vi "Setup TS.vi"(8 "error in":errorcluster, 11 "Water Tunnel Test Stand in":refnum<class "Water Tunnel Test Stand.lvclass">) -> (0 "error out":errorcluster, 3 "Water Tunnel Test Stand out":refnum<class "Water Tunnel Test Stand.lvclass">)   [LabVIEW 2019, in "Test Stands.lvlib" / "Water Tunnel Test Stand.lvclass"]
uses:
  Water Tunnel Test Stand.lvclass
  C:/Users/wg/Documents/LV_Projects/test-stand/App/Generic Test Stand/Generic Test Stand.lvclass
  DAC/Water Tunnel/Inclinometer/DAC Inclinometer.lvclass
  C:/Users/wg/Documents/LV_Projects/test-stand/App/DAC/DAC.lvclass
  DAC/Water Tunnel/Pressure Scan/DAC Pressure Scan.lvclass
  DAC/Water Tunnel/ADV/DAC ADV.lvclass
  DAC/DAC.lvclass/DAC.ctl
  Generic Test Stand/Generic Test Stand.lvclass/Generic Test Stand.ctl
  Generic Test Stand/Generic Test Stand.lvclass
  DAC/DAC.lvclass
  DAC/Water Tunnel/Traverse/DAC Traverse.lvclass
  DAC/Water Tunnel/Pump Inverter/DAC Pump Inv.lvclass
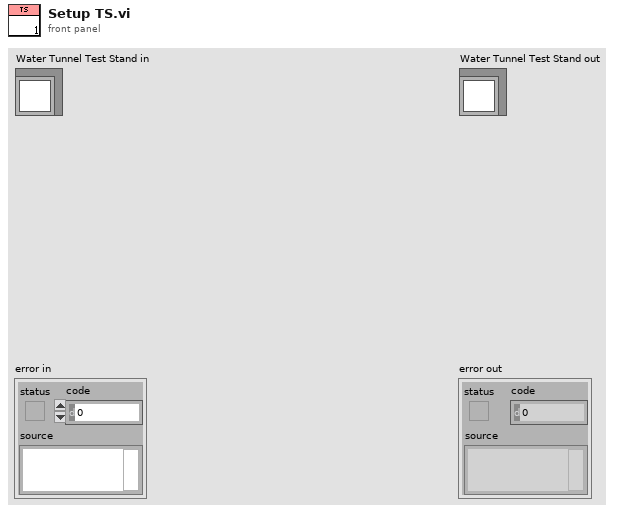
[diagram p1: front panel]
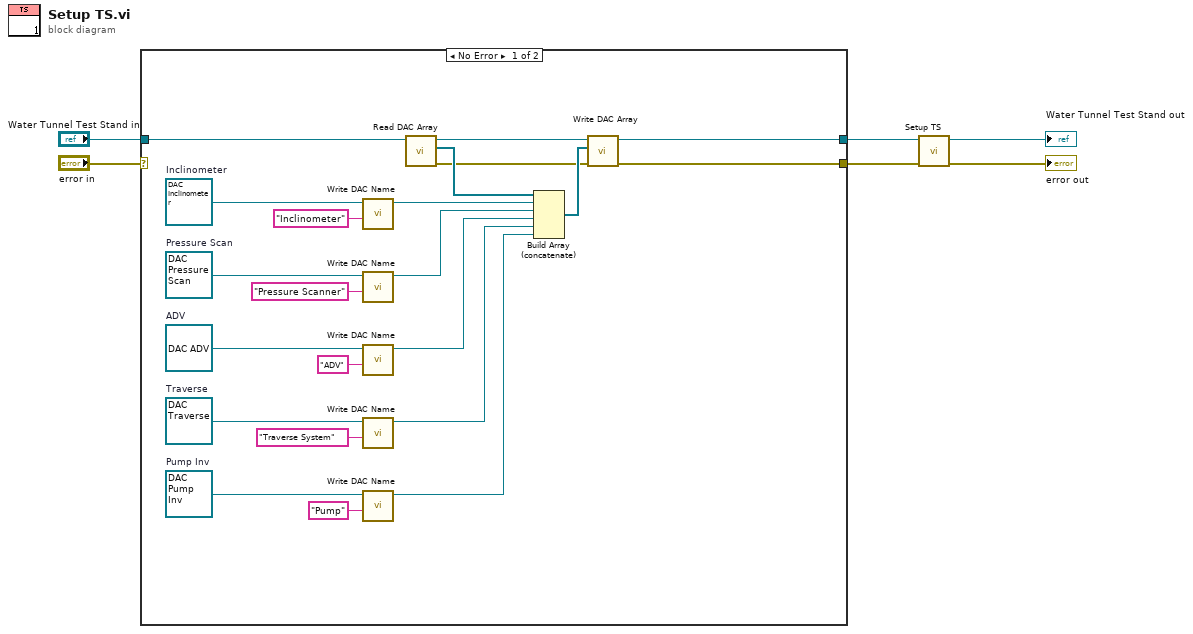
[diagram p0: block diagram]
diagram:
  n1 = case shown="No Error" "error in" {
    selector: "error in" -> [_ w29]
    tunnel: "Water Tunnel Test Stand in" -> [w28 w30]
    tunnel: [w22 w30] -> w2
    tunnel: [w21 w29] -> w1
    frame No Error {
      w9 = refnum<class "DAC Pump Inv.lvclass"> refnum  # Pump Inv
      w10 = refnum<class "DAC Traverse.lvclass"> refnum  # Traverse
      w12 = refnum<class "DAC ADV.lvclass"> refnum  # ADV
      w15 = refnum<class "DAC Pressure Scan.lvclass"> refnum  # Pressure Scan
      w16 = refnum<class "DAC Inclinometer.lvclass"> refnum  # Inclinometer
      n2 = call "Write DAC Name.vi"("DAC Name"="Inclinometer", "DAC in"=w16) -> ("DAC out"=w23:refnum<class "DAC Inclinometer.lvclass">)  [unwired: 8 in, 1 out]
      n3 = call "Write DAC Name.vi"("DAC Name"="Pressure Scanner", "DAC in"=w15) -> ("DAC out"=w13:refnum<class "DAC Pressure Scan.lvclass">)  [unwired: 8 in, 1 out]
      n4 = call "Write DAC Name.vi"("DAC Name"="ADV", "DAC in"=w12) -> ("DAC out"=w11:refnum<class "DAC ADV.lvclass">)  [unwired: 8 in, 1 out]
      n5 = call "Write DAC Name.vi"("DAC Name"="Traverse System", "DAC in"=w10) -> ("DAC out"=w8:refnum<class "DAC Traverse.lvclass">)  [unwired: 8 in, 1 out]
      n6 = call "Write DAC Name.vi"("DAC Name"="Pump", "DAC in"=w9) -> ("DAC out"=w7:refnum<class "DAC Pump Inv.lvclass">)  [unwired: 8 in, 1 out]
      n7 = call "Read DAC Array.vi"("Generic Test Stand in"=w28) -> ("error out"=w24:errorcluster, "DAC Array"=w27:refnum<class "DAC.lvclass">[], "Generic Test Stand out"=w26:refnum<class "Water Tunnel Test Stand.lvclass">)  [unwired: 8 in]
      n8 = Build Array (concatenate)(w27, w23, w13, w11, w8, w7) -> (w25:refnum<class "DAC.lvclass">[])
      n9 = call "Write DAC Array.vi"("error in (no error)"=w24, "DAC Array"=w25, "Generic Test Stand in"=w26) -> ("error out"=w21:errorcluster, "Generic Test Stand out"=w22:refnum<class "Water Tunnel Test Stand.lvclass">)  [unwired: 7 in]
    }
    frame Error {
    }
  }
  n10 = call-parent "Setup TS.vi"("error in (no error)"=w1, "Generic Test Stand in"=w2) -> ("error out"=→"error out":errorcluster, "Generic Test Stand out"=→"Water Tunnel Test Stand out":refnum<class "Water Tunnel Test Stand.lvclass">)  [unwired: 8 in]
